vi "DiffDriveSim_Read_Actuators.vi"(9 "Right Drive Motor":T1=enum."PWM 1", 10 "Left Drive Motor":T1, 11 "Robot Enabled":bool) -> (0 "Right Motor Dmd":dbl, 1 "Left Motor Dmd":dbl, 2 "Right PWM Sim":T2, 3 "Left PWM Sim":T2)   [LabVIEW 2019]
uses:
  <vilib>/Rock Robotics/WPI/Simulation/Protocol/Devices/PWM/PWM proto.ctl
  <vilib>/Rock Robotics/WPI/Simulation/Protocol/Devices/PWM/PWM data proto.ctl
  <vilib>/Rock Robotics/SystemInterfaces/DIO/FPGA_DIOPWMChannel.ctl
  <vilib>/Rock Robotics/WPI/Simulation/Protocol/Devices/PWM/PWM Update Ops.ctl
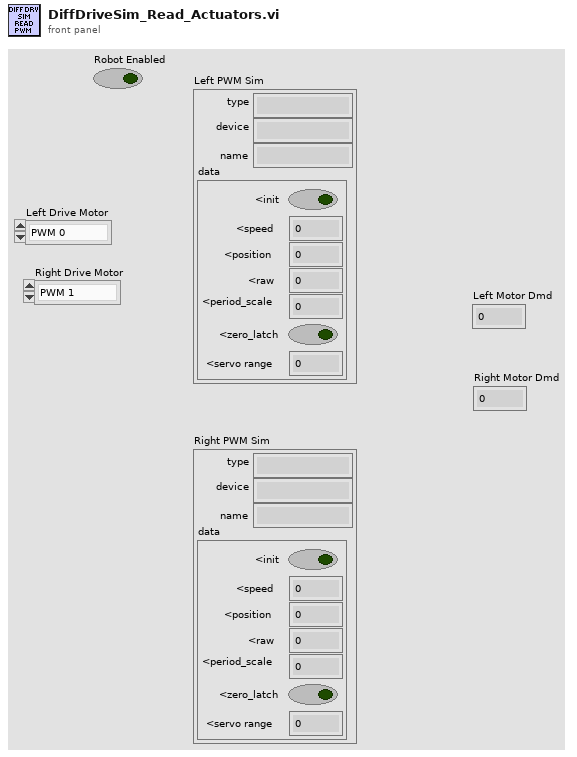
[diagram p1: front panel]
types:
  T1 = typedef "FPGA_DIOPWMChannel.ctl" = enum8{"PWM 0", "PWM 1", "PWM 2", "PWM 3", "PWM 4", "PWM 5", "PWM 6", "PWM 7", "PWM 8", "PWM 9", "PWM MXP 0", "PWM MXP 1", "PWM MXP 2", "PWM MXP 3", "PWM MXP 4", "PWM MXP 5", "PWM MXP 6", "PWM MXP 7", "PWM MXP 8", "PWM MXP 9", "Invalid"}
  T2 = typedef "PWM proto.ctl" = cluster{"type":string, "device":string, "name":string, "data":T3}
  T3 = typedef "PWM data proto.ctl" = cluster{"<init":bool, "<speed":dbl, "<position":dbl, "<raw":dbl, "<period_scale":dbl, "<zero_latch":bool, "<servo range":dbl}
  T4 = typedef "PWM Update Ops.ctl" = enum16{"set init", "set speed", "set position", "set raw", "set  period_scale", "set zero_latch", "set angular range", "get", "delete", "JSON update", "set name", "transmit initial", "reset"}
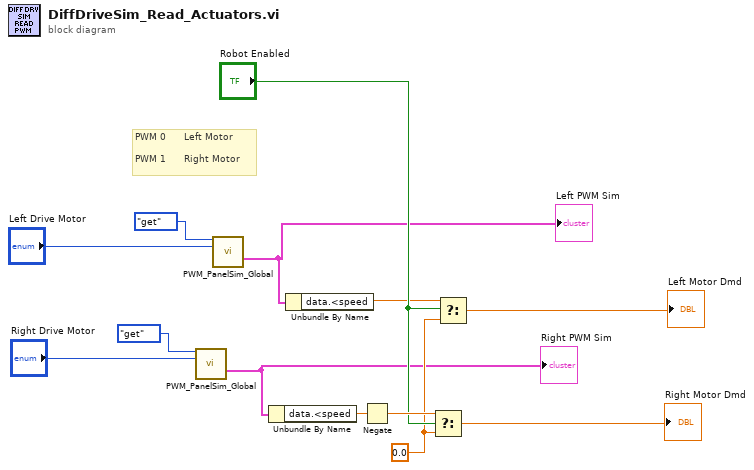
[diagram p0: block diagram]
diagram:
  w10 = 0.0 ("f")
  # "PWM 0      Left Motor\n\nPWM 1      Right Motor"
  n1 = call <vilib>:"PWM_PanelSim_Global.vi"("menu"=PWM_Update_Ops."get", "PWMChannel"="Right Drive Motor") -> ("Value get"=w6:T2)  [unwired: 12 in, 1 out]
  "Right PWM Sim" <- w6
  n2 = call <vilib>:"PWM_PanelSim_Global.vi"("menu"=PWM_Update_Ops."get", "PWMChannel"="Left Drive Motor") -> ("Value get"=w3:T2)  [unwired: 12 in, 1 out]
  "Left PWM Sim" <- w3
  n3 = Unbundle By Name(w6) -> ("data.<speed"=w12:dbl)
  n4 = Unbundle By Name(w3) -> ("data.<speed"=w9:dbl)
  n5 = Negate(x=w12) -> (-x=w13:dbl)
  n6 = Select(t=w13, s="Robot Enabled", f=w10) -> (s? t:f=→"Right Motor Dmd":dbl)
  n7 = Select(t=w9, s="Robot Enabled", f=w10) -> (s? t:f=→"Left Motor Dmd":dbl)
